vi "IMAQController.SaveImage.vi"(0 "Image":T3, 1 "Save path in":path, 2 "Service name":string, 3 "Save?":bool, 4 "Save Overlay?":bool, 5 "error in":errorcluster, 6 "Aqcuisation Mode":T2(ring), 7 "User Palette":cluster{"Red":u8, "Green":u8, "Blue":u8}[](array[cluster]), 9 "Color Palette":cluster{"Red":u8, "Green":u8, "Blue":u8}[](array[cluster]), 11 "Scan Variables":T1, 13 "Scan Running?":bool) -> (14 "Save path out Scan folder":path, 15 "Save path out Horizontal":path, 17 "Save path out Verical":path, 19 "error out":errorcluster)   [LabVIEW 2014, in "IMAQController.lvlib"]
uses:
  IMAQController.lvlib
  <vilib>/vision/Image Controls.llb/IMAQ Image.ctl
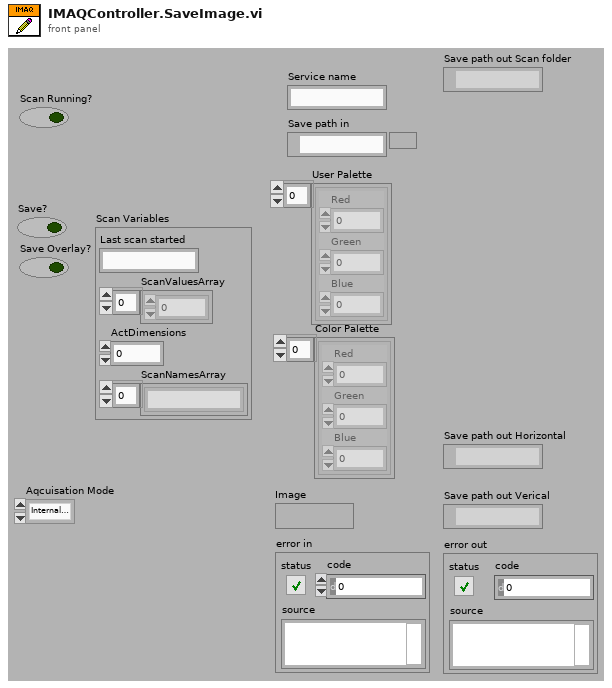
[diagram p1: front panel]
types:
  T1 = cluster{"Last scan started":string, "ScanValuesArray":dbl[], "ActDimensions":i16, "ScanNamesArray":string[]}
  T2 = enum32{"Internal Trigger", "Scan", "free Running", "External Trigger"}
  T3 = typedef "IMAQ Image.ctl" = refnum<image>
  T4 = typedef "Image Type" = u32
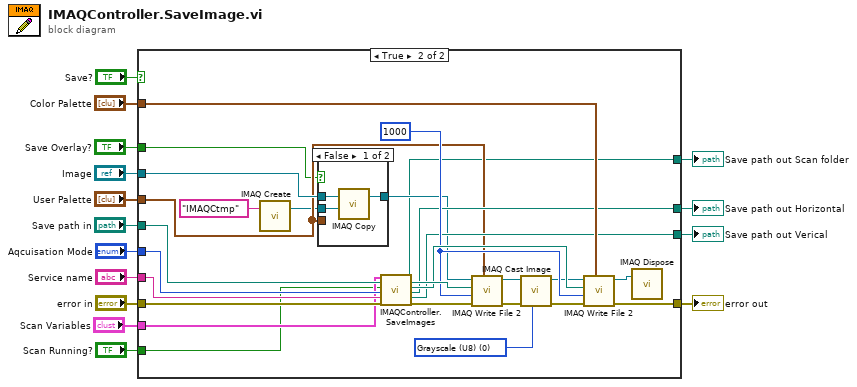
[diagram p0: block diagram]
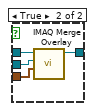
[diagram p3: hidden frame]
diagram:
  n1 = case shown="True" "Save?" {
    tunnel: "error in" -> [w17 w31]
    tunnel: [w17 w29] -> w15
    tunnel: "Image" -> [_ w34]
    tunnel: "User Palette" -> [_ w32]
    tunnel: "Service name" -> [_ w43]
    tunnel: "Color Palette" -> [_ w40]
    tunnel: "Save path in" -> [w16 w39]
    tunnel: "Aqcuisation Mode" -> [_ w38]
    tunnel: [w16 w36] -> w13
    tunnel: [w16 w35] -> w14
    tunnel: "Save Overlay?" -> [_ w21]
    tunnel: "Scan Variables" -> [_ w20]
    tunnel: [w16 w19] -> w3
    tunnel: "Scan Running?" -> [_ w18]
    frame False {
    }
    frame True {
      w26 = T4 0 items=["Grayscale (U8)", "Grayscale (I16)", "Grayscale (SGL)", "Complex (CSG)", "RGB (U32)", "HSL (U32)", "RGB (U64)"] ("Image Type")
      w37 = u32 1000 ("Image Quality")
      n2 = call "IMAQ Create"("Image Name"="IMAQCtmp") -> ("New Image"=w30:T3)  [unwired: 4 in, 1 out]
      n3 = case shown="False" w21 {
        tunnel: w34 -> [w46 w51]
        tunnel: [w47 w50] -> w33
        tunnel: w32 -> [_ w49]
        tunnel: w30 -> [w45 w48]
        frame False {
          n4 = call "IMAQ Copy"("Image Dst"=w45, "Image Src"=w46) -> ("Image Dst Out"=w47:T3)  [unwired: 4 in, 1 out]
        }
        frame True {
          n5 = call "IMAQ Merge Overlay"("Color Palette"=w49, "Image Dst"=w48, "Image Src"=w51) -> ("Image Dst Out"=w50:T3)  [unwired: 7 in, 1 out]
        }
      }
      n6 = call "IMAQController.SaveImages.vi"("Scan Variables"=w20, "Save path in"=w39, "Scan running?"=w18, "Acquisition Mode"=w38, "serviceName"=w43, "error in (no error)"=w31) -> ("Save path out Scan folder"=w19:path, "Save path out Rainbow"=w42:path, "Save path out Original"=w41:path, "Save path out Horizontal"=w36:path, "Save path out Verical"=w35:path, "error out"=w44:errorcluster)  [unwired: 8 in]
      n7 = call-poly "IMAQ Write File 2"("Color Palette"=w32, "error in (no error)"=w44, "Image Quality"=w37, "File Path"=w42, "Image"=w33) -> ("error out"=w23:errorcluster, "Image Out (duplicate)"=w25:T3)  [unwired: 5 in]
      n8 = call "IMAQ Cast Image"("Image Type"=w26, "error in (no error)"=w23, "Image Src"=w25) -> ("error out"=w22:errorcluster, "Image Dst Out"=w24:T3)  [unwired: 7 in]
      n9 = call-poly "IMAQ Write File 2"("Color Palette"=w40, "error in (no error)"=w22, "Image Quality"=w37, "File Path"=w41, "Image"=w24) -> ("error out"=w29:errorcluster, "Image Out (duplicate)"=w28:T3)  [unwired: 5 in]
      n10 = call "IMAQ Dispose"("Image"=w28) -> ()  [unwired: 5 in, 1 out]
    }
  }
  "error out" <- w15
  "Save path out Verical" <- w14
  "Save path out Horizontal" <- w13
  "Save path out Scan folder" <- w3
